vi "create cipher context.vi"(8 "error in":errorcluster) -> (0 "error out":errorcluster, 3 "lvlibcrypto digest out":refnum<class "lvlibcrypto cipher.lvclass">)   [LabVIEW 2016, in "lvlibcrypto cipher.lvclass"]
uses:
  lvlibcrypto cipher.lvclass
  lvlibcrypto cipher.lvclass/lvlibcrypto cipher.ctl
  lv tls dll.lvlib
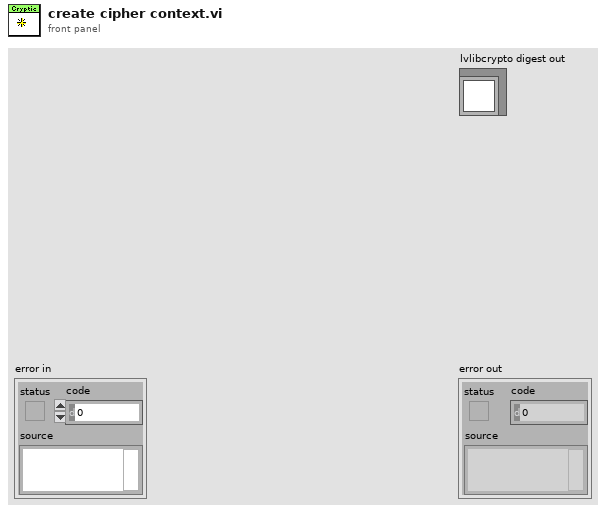
[diagram p1: front panel]
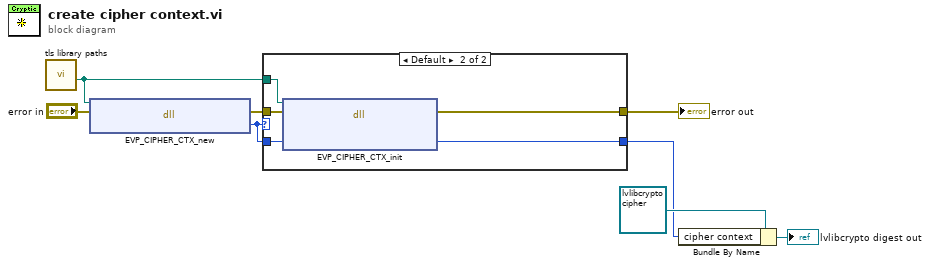
[diagram p0: block diagram]
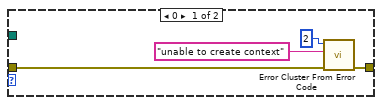
[diagram p2: hidden frame]
diagram:
  n1 = call "tls library paths.vi"() -> ("libcrypto"=w3:path)  [unwired: 8 in, 3 out]
  n2 = dll-call lib="C:/Users/IEUser/Desktop/tlssimple/libcrypto-41.dll" fn="EVP_CIPHER_CTX_new"(path in=w3, error in="error in") -> (error out=w2:errorcluster, "context"=w1:u64)  [unwired: 1 in, 1 out]
  n3 = case shown="Default" w1 {
    tunnel: w2 -> [w12 w17]
    tunnel: [w11 w16] -> w6
    tunnel: w1 -> [_ w14]
    tunnel: w3 -> [_ w15]
    tunnel: [_ w13] -> w4
    frame 0 {
      n4 = call <vilib>:"Error Cluster From Error Code.vi"("error in (no error)"=w12, "error message (\"\")"="unable to create context" ("error message (\"\")"), "error code (0)"=2) -> ("error out"=w11:errorcluster)  [unwired: 6 in]
    }
    frame Default {
      n5 = dll-call lib="C:/Users/IEUser/Desktop/tlssimple/libcrypto-41.dll" fn="EVP_CIPHER_CTX_init"(path in=w15, error in=w17, "context"=w14) -> (error out=w16:errorcluster, "context"=w13:u64)  [unwired: 2 in, 1 out]
    }
  }
  "error out" <- w6
  n6 = Bundle By Name(cluster=refnum<class "lvlibcrypto cipher.lvclass"> refnum ("lvlibcrypto digest in"), "cipher context"=w4) -> (→"lvlibcrypto digest out":refnum<class "lvlibcrypto cipher.lvclass">)
